vi "Mass Compile LabVIEW Tool.vi"(7 "Only Check Launcher? (F: Check Entire Product)":bool, 8 "error in (no error)":errorcluster, 10 "Product Folders":path[](array[path]), 11 "Product Name":string) -> (0 "error out":errorcluster, 2 "User Aborted?":bool)   [LabVIEW 2020]
doc: "This VI self-mass compiles an installed LabVIEW Tool. It should be run by a tool, during its start-up process."
panel:
  # "Copyright © 2006-2011 JKI. All rights reserved.\n\nAuthor: Jim Kring <jim.kring@jki.net>\n\nThis library is provided \"AS IS\" , WITHOUT WARRANTIES OR \nCONDITIONS OF ANY KIND, either express or implied.\n\nJKI -- jki.net"
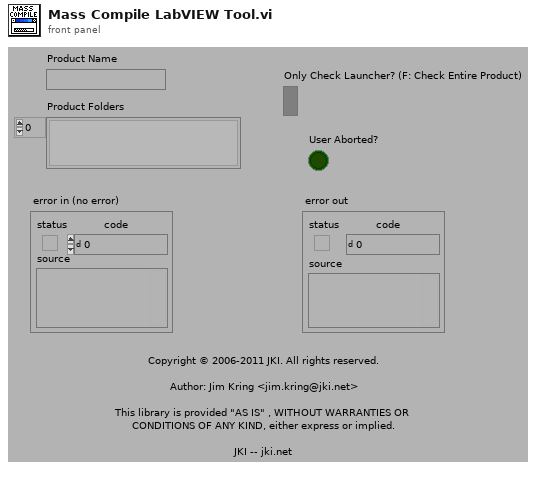
[diagram p1: front panel]
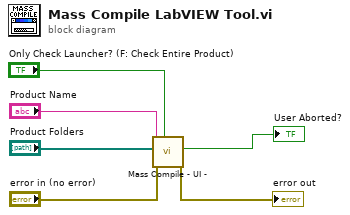
[diagram p0: block diagram]
diagram:
  n1 = call "Mass Compile - UI - .vi"("Only Check Launcher? (F: Check Entire Product)"="Only Check Launcher? (F: Check Entire Product)", "error in (no error)"="error in (no error)", "Product Folders"="Product Folders", "Product Name"="Product Name") -> ("error out"=→"error out":errorcluster, "User Aborted?"=→"User Aborted?":bool)  [unwired: 6 in]
